vi "Set UI Interaction.vi"(8 "error in (no error)":errorcluster {"code" format="Error %.0f"}, 10 "UI Interaction":refnum<class "UI Interaction.lvclass">, 11 "VIDoc Parser In":refnum<class "VIDoc Parser.lvclass">) -> (0 "error out":errorcluster {"code" format="Error %.0f"}, 3 "VIDoc Parser Out":refnum<class "VIDoc Parser.lvclass">)   [LabVIEW 2023, in "VIDoc Parsing.lvlib" / "VIDoc Parser.lvclass"]
uses:
  VIDoc Parser.lvclass
  VIDoc Parser.lvclass/VIDoc Parser.ctl
  UI Interaction/Interface/UI Interaction.lvclass
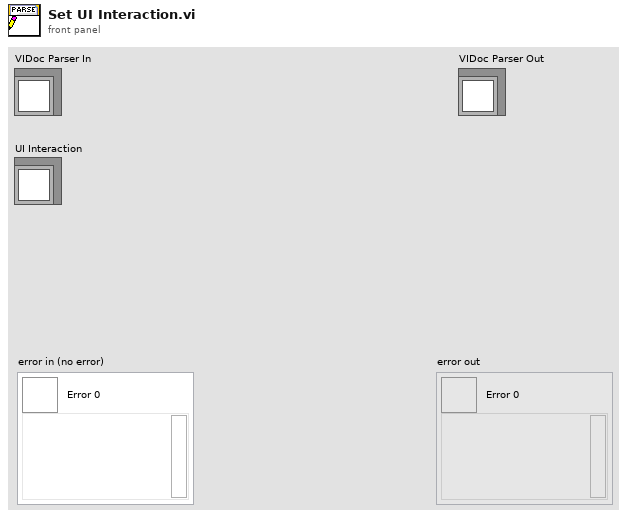
[diagram p1: front panel]
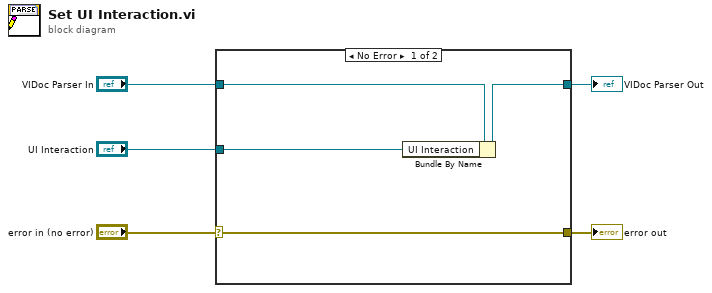
[diagram p0: block diagram]
diagram:
  n1 = case shown="No Error" "error in (no error)" {
    selector: "error in (no error)" -> [w9 w10]
    tunnel: [w9 w10] -> w4
    tunnel: [w7 w11] -> w2
    tunnel: "VIDoc Parser In" -> [w8 w11]
    tunnel: "UI Interaction" -> [w6 _]
    frame No Error {
      n2 = Bundle By Name(cluster=w8, "UI Interaction"=w6) -> (w7:refnum<class "VIDoc Parser.lvclass">)
    }
    frame Error {
    }
  }
  "error out" <- w4
  "VIDoc Parser Out" <- w2
